vi "Do Deinitialize.vi"(8 "error in (no error)":errorcluster, 11 "Output Actor Hardware in":refnum<class "Output Actor Hardware.lvclass">) -> (0 "error out":errorcluster, 3 "Output Actor Hardware out":refnum<class "Output Actor Hardware.lvclass">)   [LabVIEW 2015, in "Output Actor Hardware.lvclass"]
uses:
  Output Actor Hardware.lvclass
  state.ctl
  Output Actor Hardware.lvclass/Output Actor Hardware.ctl
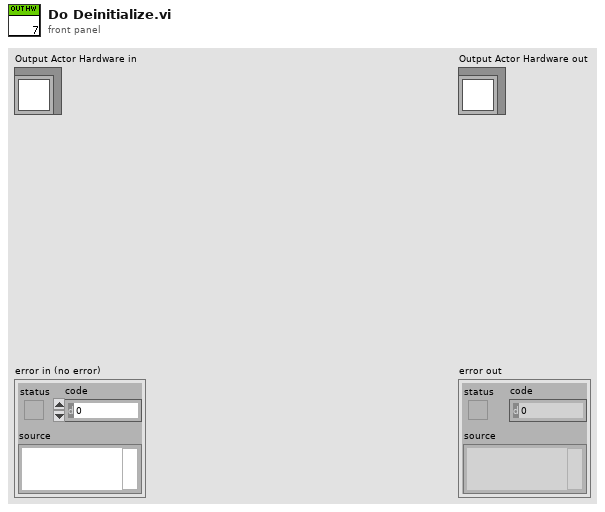
[diagram p1: front panel]
types:
  T1 = typedef "Output Actor Hardware.lvclass/state.ctl" = enum16{"not_available", "not_initialized", "ok"}
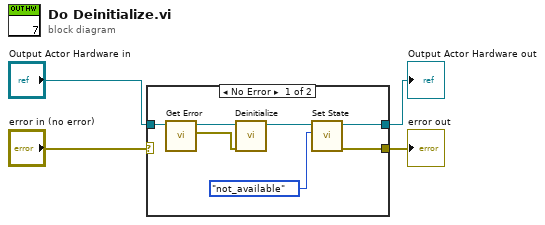
[diagram p0: block diagram]
diagram:
  n1 = case shown="No Error" "error in (no error)" {
    selector: "error in (no error)" -> [_ w13]
    tunnel: [w6 w13] -> w3
    tunnel: [w5 w12] -> w1
    tunnel: "Output Actor Hardware in" -> [w9 w12]
    frame No Error {
      n2 = call "Get Error.vi"("Output Actor Hardware in"=w9) -> ("Error"=w11:errorcluster, "Output Actor Hardware out"=w10:refnum<class "Output Actor Hardware.lvclass">)  [unwired: 8 in, 1 out]
      n3 = call-dynamic "Deinitialize.vi"("error in (no error)"=w11, "Output Actor Hardware in"=w10) -> ("Output Actor Hardware out"=w8:refnum<class "Output Actor Hardware.lvclass">)  [unwired: 9 in]
      n4 = call "Set State.vi"("state"=state."not_available", "output_actor_errorneous in"=w8) -> ("error out"=w6:errorcluster, "output_actor_errorneous out"=w5:refnum<class "Output Actor Hardware.lvclass">)  [unwired: 8 in]
    }
    frame Error {
    }
  }
  "error out" <- w3
  "Output Actor Hardware out" <- w1
